vi "Oritentation Global.vi"() -> ()   [LabVIEW 2013]
panel:
  in  "Scaling Factor Camera Mounted (V/M)":dbl
  in  "Scaling Factor Rear (V/M)":dbl
  in  "Scaling Factor Front Left (V/M)":dbl
  in  "Scaling Factor Front Right (V/M)":dbl
  in  "Distance Between Front Sensors":dbl
  in  "Oriantation Info":T1
  # "The Horizontal \nVector of the \nCamera Mounts\nDistance"
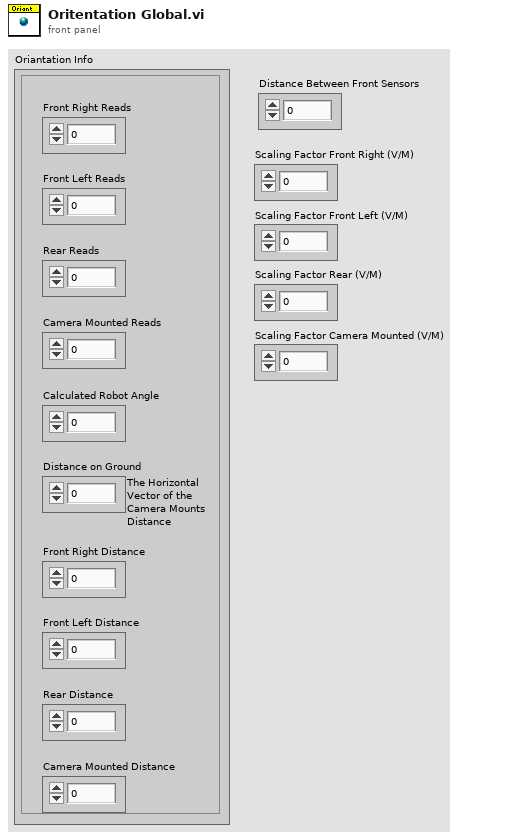
[diagram p1: front panel]
types:
  T1 = cluster{"Front Right Reads":dbl, "Front Left Reads ":dbl, "Rear Reads":dbl, "Camera Mounted Reads":dbl, "Calculated Robot Angle":dbl, "Distance on Ground":dbl, "Front Right Distance":dbl, "Front Left Distance":dbl, "Rear Distance":dbl, "Camera Mounted Distance":dbl}
diagram:
